vi "Initialise GUI.vi"(8 "error in":errorcluster, 11 "Main GUI VI Reference In":refnum<vi>) -> (0 "error out":errorcluster)   [LabVIEW 2017, in "DTacq Plot Display Library.lvlib"]
doc: "Prepares the graphical user interface for display;\nGUI controls are set to their default values,\nThe front panel is centered on the screen,\nThe front panel is opened, if not already open"
uses:
  DTacq Plot Display Library.lvlib
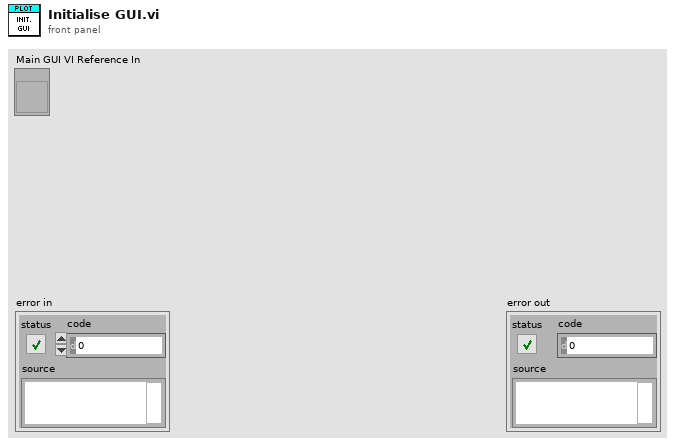
[diagram p1: front panel]
types:
  T1 = enum32{"Invalid", "Standard", "Closed", "Hidden", "Minimized", "Maximized"}
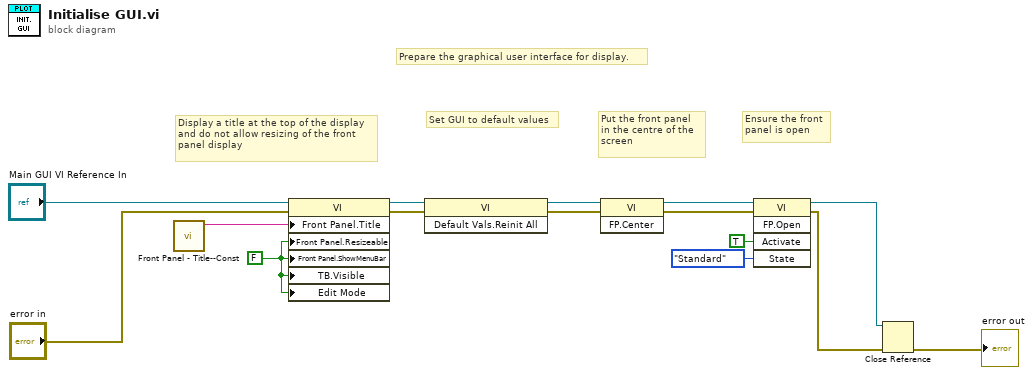
[diagram p0: block diagram]
diagram:
  w4 = FALSE ("Front Panel Window:Show Menu Bar")
  # "Display a title at the top of the display\nand do not allow resizing of the front\npanel display"
  # "Prepare the graphical user interface for display."
  # "Ensure the front\npanel is open"
  # "Put the front panel\nin the centre of the \nscreen"
  # "Set GUI to default values"
  n1 = call "Front Panel - Title--Const.vi"() -> ("Window Title"=w6:string)  [unwired: 11 in]
  n2 = property class="VI"(reference="Main GUI VI Reference In", error in="error in", "Front Panel.Title"=w6, "Front Panel.Resizeable"=w4, "Front Panel.ShowMenuBar"=w4, "TB.Visible"=w4, "Edit Mode"=w4) -> (reference out=w7:refnum<vi>, error out=w8:errorcluster)
  n3 = invoke class="VI" method="Default Vals.Reinit All"(reference=w7, error in=w8) -> (reference out=w13:refnum<vi>, error out=w12:errorcluster)  [unwired: 1 in, 1 out]
  n4 = invoke class="VI" method="FP.Center"(reference=w13, error in=w12) -> (reference out=w11:refnum<vi>, error out=w10:errorcluster)  [unwired: 1 in, 1 out]
  n5 = invoke class="VI" method="FP.Open"(reference=w11, error in=w10, "Activate"=TRUE ("Activate?"), "State"=T1."Standard") -> (reference out=w2:refnum<vi>, error out=w1:errorcluster)  [unwired: 1 in, 3 out]
  n6 = Close Reference(reference=w2, error in (no error)=w1) -> (error out=→"error out":errorcluster)
